vi "checkChecksum.vi"(8 "error in (no error)":errorcluster, 10 "TPDO data":u8[](array[numeric]), 11 "Orion_BMS in":refnum<class "Orion_BMS.lvclass">) -> (0 "error out":errorcluster, 2 "checkSumMatched":bool, 3 "Orion_BMS out":refnum<class "Orion_BMS.lvclass">)   [LabVIEW 2017, in "Orion_BMS.lvclass"]
uses:
  Orion_BMS.lvclass
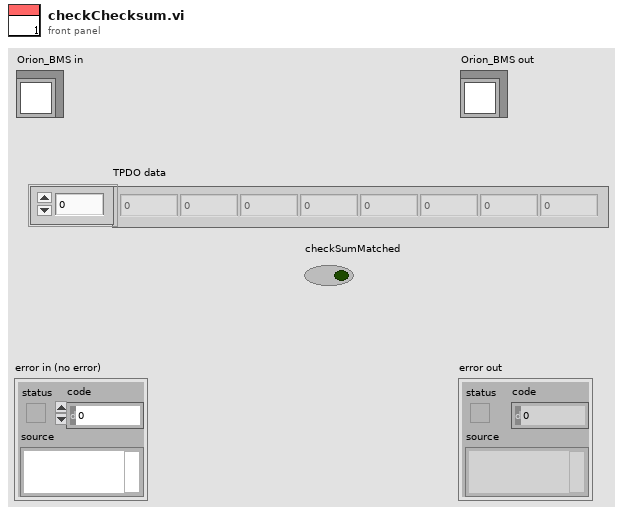
[diagram p1: front panel]
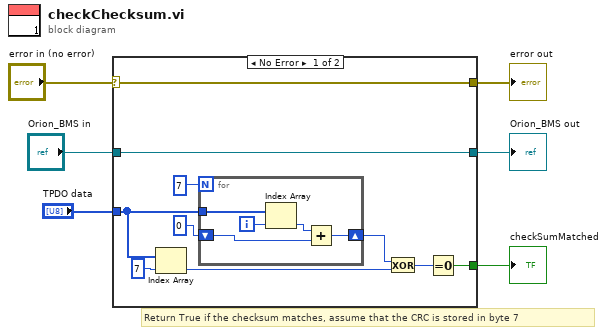
[diagram p0: block diagram]
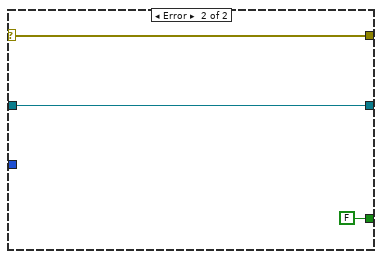
[diagram p2: hidden frame]
diagram:
  # "Return True if the checksum matches, assume that the CRC is stored in byte 7"
  n1 = case shown="No Error" "error in (no error)" {
    selector: "error in (no error)" -> [w8 w24]
    tunnel: [w8 w24] -> w5
    tunnel: [w16 w23] -> w3
    tunnel: "Orion_BMS in" -> [w16 w23]
    tunnel: [w13 FALSE ("Boolean")] -> w1
    tunnel: "TPDO data" -> [w11 _]
    frame No Error {
      n2 = Index Array(array=w11, index=7) -> (element=w14:u8)
      n3 = for {
        N: 7 -> [_]
        tunnel: w11 -> [w21]
        shift-right: [w18] -> w7
        shift-left: u8 0 -> [w17]
        i -> [w20]
        n4 = Index Array(array=w21, index=w20) -> (element=w19:u8)
        n5 = Add(x=w19, y=w17) -> (x+y=w18:u8)
      }
      n6 = Exclusive Or(1:w14, 2:w7) -> (0:w9:u8)
      n7 = Equal To 0?(x=w9) -> (x = 0?=w13:bool)
    }
    frame Error {
    }
  }
  "error out" <- w5
  "Orion_BMS out" <- w3
  "checkSumMatched" <- w1
